vi "Autotest.vi"(8 "error in (no error)":errorcluster caption="entrée d'erreur (pas d'erreur)", 11 "Class Printer_CAB en entrée":refnum<class "Class Printer_CAB.lvclass">) -> (0 "error out":errorcluster caption="sortie d'erreur", 2 "Autotest Ok ?":bool, 3 "Class Printer_CAB en sortie":refnum<class "Class Printer_CAB.lvclass">)   [LabVIEW 2020, in "Library Instrument & Equipement.lvlib" / "Library Printer.lvlib" / "Class Printer_CAB.lvclass"]
uses:
  Class Printer_CAB.lvclass
  C:/Users/ngarcin/OneDrive - Altyor/Standard TB/Class/Printer/Printer (Default)/Class Printer (Default).lvclass
  <vilib>/Instr/_visa.llb/VISA Find Search Mode.ctl
  Printer (Default)/Class Printer (Default).lvclass
  Class Printer_CAB.lvclass/Class Printer_CAB.ctl
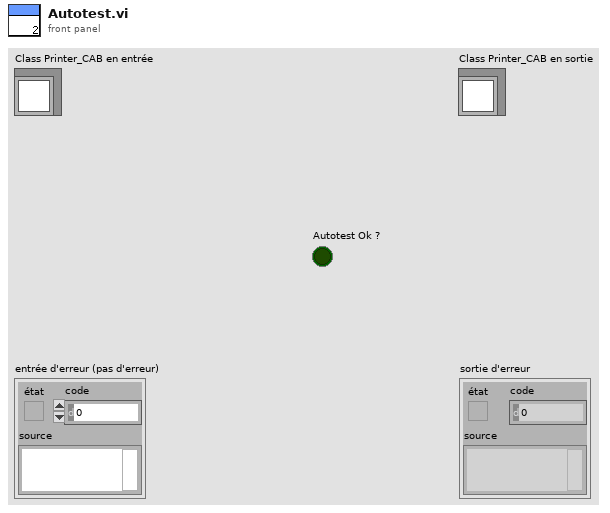
[diagram p1: front panel]
types:
  T1 = typedef "VISA Find Search Mode.ctl" = u32
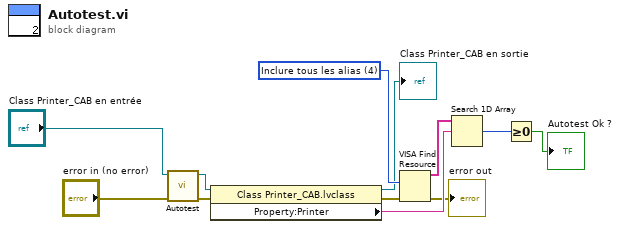
[diagram p0: block diagram]
diagram:
  w9 = T1 4 items=["Noms canoniques uniquement"=0, "Alias uniquement"=2, "Inclure les alias correspondants"=3, "Inclure tous les alias"=4] ("Search Mode")
  n1 = call-parent "Autotest.vi"("error in (no error)"="error in (no error)", "Class Printer (Default) en entrée"="Class Printer_CAB en entrée") -> ("error out"=w2:errorcluster, "Class Printer (Default) en sortie"=w5:refnum<class "Class Printer_CAB.lvclass">)  [unwired: 7 in, 1 out]
  n2 = property class="Class Printer_CAB.lvclass"(reference=w5, error in=w2) -> (reference out=→"Class Printer_CAB en sortie":refnum<class "Class Printer_CAB.lvclass">, error out=w10:errorcluster, "Property:Printer"=w8:string)
  n3 = VISA Find Resource(8:w10, 10:w9) -> (0:→"error out":errorcluster, 3:w7:string[])  [unwired: 1 in, 1 out]
  n4 = Search 1D Array(1D array=w7, element=w8) -> (index of element=w6:i32)  [unwired: 1 in]
  n5 = Greater Or Equal To 0?(x=w6) -> (x >= 0?=→"Autotest Ok ?":bool)
